vi "Vertical Red Dot Not.vi"(2 "B":bool) -> (7 "Not(B)":bool)   [LabVIEW 2021, in "Boolean.lvlib"]
uses:
  Boolean.lvlib
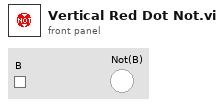
[diagram p1: front panel]
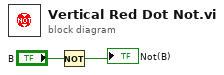
[diagram p0: block diagram]
diagram:
  n1 = Not(x="B") -> (.not. x?=→"Not(B)":bool)
